vi "ManipGroundPickup.vi"(2 "Reinit":bool, 3 "Parameter String":string) -> (0 "error out":errorcluster, 1 "Advance Trigger":bool)   [LabVIEW 2020]
doc: "This VI commands the robot to pick a game piece off of the ground while in the GROUND state.\n\nParameters:\nDecides turn the gripper on or off"
uses:
  SafeParser_String.vi
  GlobalDriverStationCommands.vi
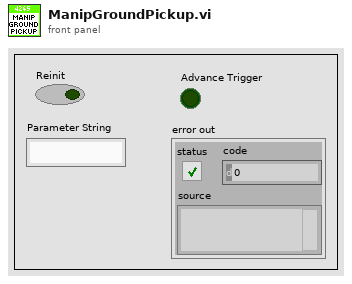
[diagram p1: front panel]
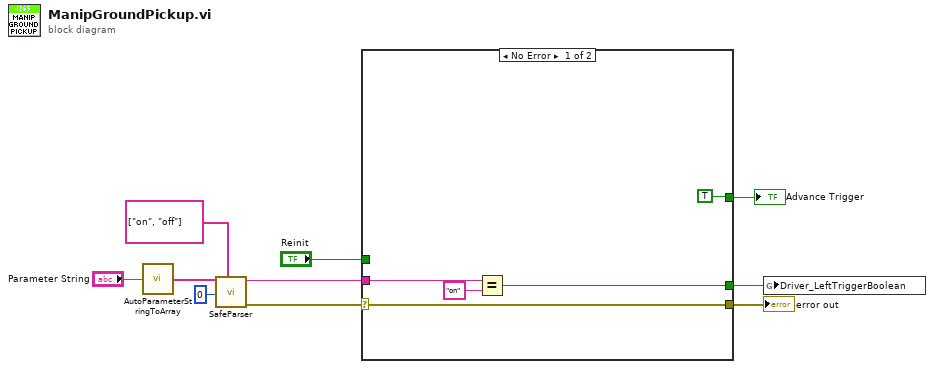
[diagram p0: block diagram]
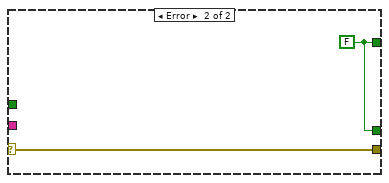
[diagram p2: hidden frame]
diagram:
  n1 = call "AutoParameterStringToArray.vi"("Parameter String"="Parameter String") -> ("Parsed Parameters"=w8:string[])
  n2 = call-poly "SafeParser.vi"("Allowed Values"=string[] ["on", "off"], "Array Index"=0 ("Parameter Index"), "String Array"=w8) -> ("Error Out"=w6:errorcluster, "Typecast Value"=w4:string)  [unwired: 7 in]
  n3 = case shown="No Error" w6 {
    selector: w6 -> [w15 w17]
    tunnel: [w11 w16] -> w1
    tunnel: [w15 w17] -> w5
    tunnel: w4 -> [w14 _]
    tunnel: [TRUE w16] -> w3
    tunnel: "Reinit" -> [_ _]
    frame No Error {
      n4 = Equal?(x=w14, y="on") -> (x = y?=w11:bool)
    }
    frame Error {
      w16 = FALSE
    }
  }
  "Advance Trigger" <- w3
  "error out" <- w5
  n5 = global write "GlobalDriverStationCommands.vi" "Driver_LeftTriggerBoolean"(w1) -> ()
